vi "AnalyzePulseTrain for PulseGuard.vi"(0 "Waveform In":waveform(dbl)={"t0"=timestamp(3433165898.5470004 s since 1904-01-01), "dt"=1e-05, "Y"=array[4250 elements]}, 5 "Repetitions in the Input Waveform":i32, 7 "Pulse Characteristics":T1={"Pulses per Cycle"=2, "Load Resistance (Ohms)"=750.0, "Krec Value"=2, "Recovery Mode (T=Active)"=TRUE, "Target Stim Currents (Amps)"=[]}) -> (2 "Last Pulse Width":dbl format="%0.2f", 4 "Number of Pulses Found":i32, 8 "Last Pulse Amplitude":dbl format="%0.2f")   [LabVIEW 2010]
uses:
  <vilib>/measure/mamon.llb/Trigger Detection for 1 Channel.vi
  <vilib>/measure/NI_MAPro.lvlib
  <vilib>/Analysis/NI_AALBase.lvlib
panel:
  out "Normalized Waveform":waveform(dbl)(graph)
  # "The input waveform should be a capture of the STIM chip output\n(before the cap) when the output is held at 1/2 HVDD by the\nLoad Resistance.  This ensures that passive recovery and CBC\npulses are captured, because they look like pulses pulled to GND."
  # "The elements in these arrays correspond to the pulses per cycle.\nThey are the averages over all the repetitions in the waveform."
  # "Enter Target Current\nfor each in array below"
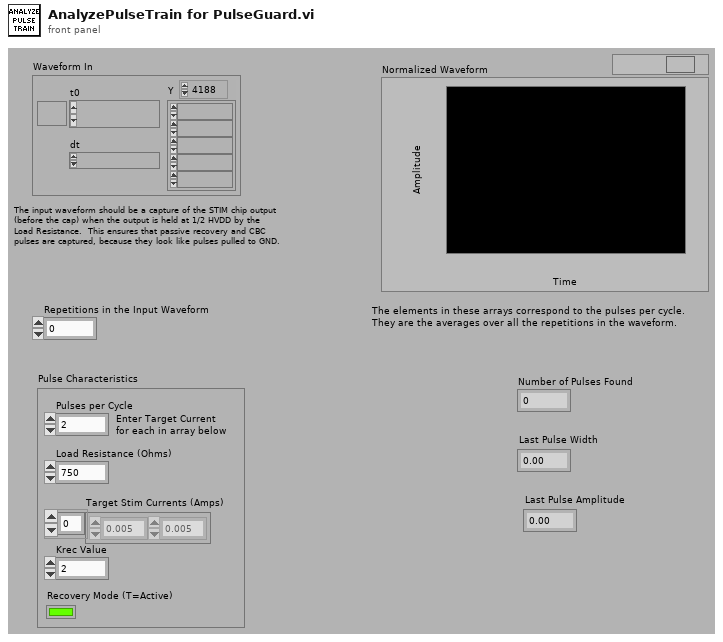
[diagram p1: front panel]
types:
  T1 = cluster{"Pulses per Cycle":i32, "Load Resistance (Ohms)":dbl, "Krec Value":i32, "Recovery Mode (T=Active)":bool, "Target Stim Currents (Amps)":dbl[]}
  T2 = cluster{"trigger slope":u16, "Trigger Level":dbl}[]
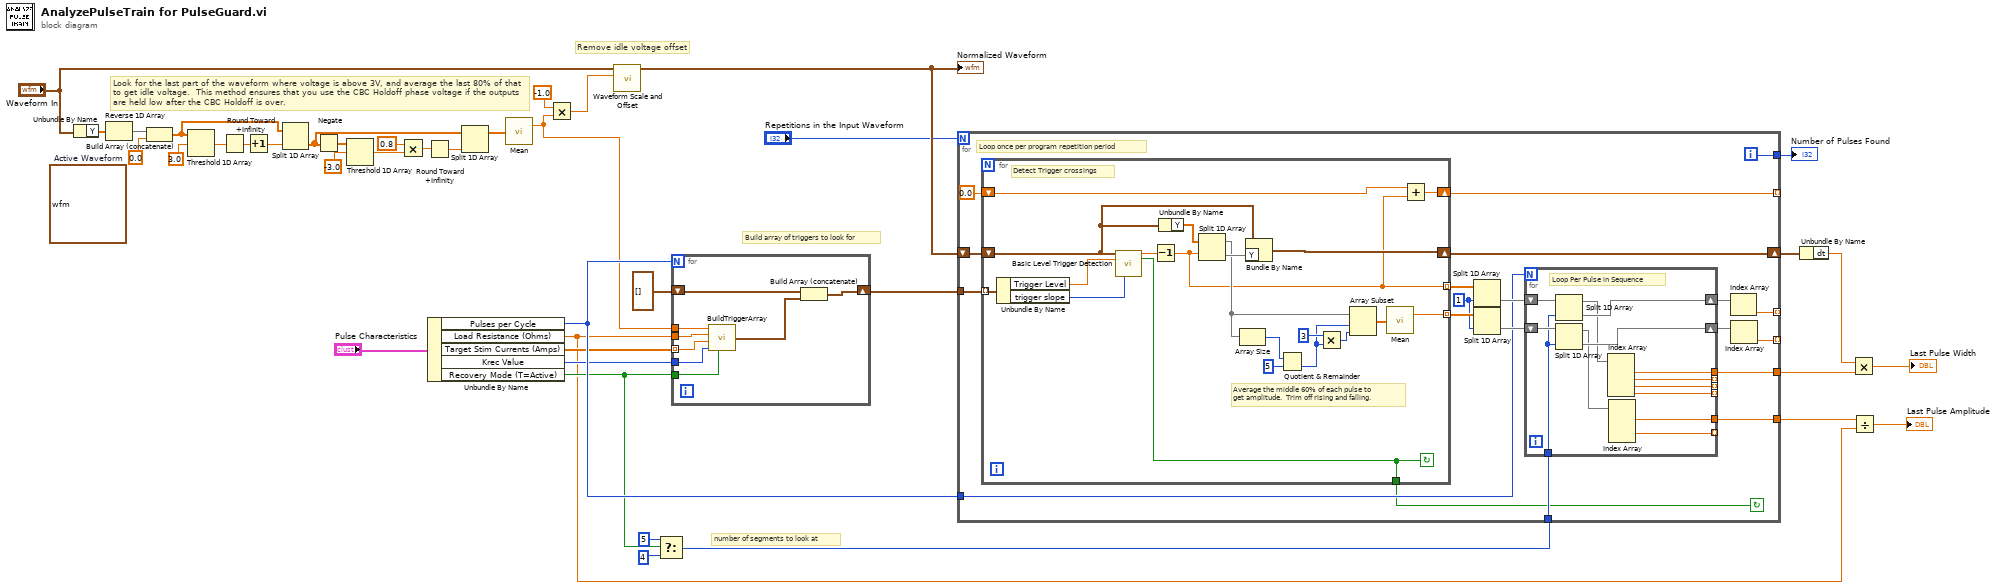
[diagram p0: block diagram]
diagram:
  (unwired) waveform(dbl) {"t0"=timestamp(3418839276.250478 s since 1904-01-01), "dt"=1e-06, "Y"=[5.0, 5.0, 9.0, 9.0, 9.0, 9.0, 9.0, 9.0, 9.0, 9.0, 5.0, 5.0, 5.0, 3.0, 3.0, 3.0, 3.0, 3.0, 3.0, 3.0, 3.0, 3.0, 3.0, 3.0, 3.0, 3.0, 3.0, 3.0, 3.0, 5.0, 5.0, 5.0, 5.0, 8.0, 8.0, 8.0, 8.0, 8.0, 8.0, 8.0, 8.0, 5.0, 5.0, 5.0, 3.0, 3.0, 3.0, 3.0, 3.0, 3.0, 3.0, 3.0, 3.0, 3.0, 3.0, 3.0, 3.0, 3.0, 3.0, 3.0, 5.0, 5.0, 5.0, 5.0, 0.0, 0.0, 0.0, 0.0, 0.0, 5.0, 5.0, 5.0, 5.0, 5.0, 5.0, 5.0, 5.0, 5.0, 5.0, 5.0, 5.0, 5.0, 5.0, 5.0, 5.0, 5.0, 5.0, 5.0, 5.0, 5.0, 5.0, 5.0, 5.0, 5.0, 5.0, 5.0, 5.0, 5.0, 5.0, 5.0, 5.0, 5.0, 9.0, 9.0, 9.0, 9.0, 9.0, 9.0, 9.0, 9.0, 5.0, 5.0, 5.0, 3.0, 3.0, 3.0, 3.0, 3.0, 3.0, 3.0, 3.0, 3.0, 3.0, 3.0, 3.0, 3.0, 3.0, 3.0, 3.0, 5.0, 5.0, 5.0, 5.0, 8.0, 8.0, 8.0, 8.0, 8.0, 8.0, 8.0, 8.0, 5.0, 5.0, 5.0, 3.0, 3.0, 3.0, 3.0, 3.0, 3.0, 3.0, 3.0, 3.0, 3.0, 3.0, 3.0, 3.0, 3.0, 3.0, 3.0, 5.0, 5.0, 5.0, 5.0, 0.0, 0.0, 0.0, 0.0, 0.0, 5.0, 5.0, 5.0, 5.0, 5.0, 5.0, 5.0, 5.0, 5.0, 5.0, 5.0, 5.0, 5.0, 5.0, 5.0, 5.0, 5.0, 5.0, 5.0, 5.0, 5.0, 5.0, 5.0, 5.0, 5.0, 5.0, 5.0, 5.0, 5.0, 5.0, 5.0, 5.0, 5.0, 9.0, 9.0, 9.0, 9.0, 9.0, 9.0, 9.0, 9.0, 5.0, 5.0, 5.0, 3.0, 3.0, 3.0, 3.0, 3.0, 3.0, 3.0, 3.0, 3.0, 3.0, 3.0, 3.0, 3.0, 3.0, 3.0, 3.0, 5.0, 5.0, 5.0, 5.0, 8.0, 8.0, 8.0, 8.0, 8.0, 8.0, 8.0, 8.0, 5.0, 5.0, 5.0, 3.0, 3.0, 3.0, 3.0, 3.0, 3.0, 3.0, 3.0, 3.0, 3.0, 3.0, 3.0, 3.0, 3.0, 3.0, 3.0, 5.0, 5.0, 5.0, 5.0, 0.0, 0.0, 0.0, 0.0, 0.0, 5.0, 5.0, 5.0, 5.0, 5.0, 5.0, 5.0, 5.0, 5.0, 5.0, 5.0, 5.0, 5.0, 5.0, 5.0, 5.0, 5.0, 5.0, 5.0, 5.0, 5.0, 5.0, 5.0, 5.0, 5.0, 5.0, 5.0, 5.0, 5.0, 5.0, 5.0, 5.0, 5.0, 9.0, 9.0, 9.0, 9.0, 9.0, 9.0, 9.0, 9.0, 5.0, 5.0, 5.0, 3.0, 3.0, 3.0, 3.0, 3.0, 3.0, 3.0, 3.0, 3.0, 3.0, 3.0, 3.0, 3.0, 3.0, 3.0, 3.0, 5.0, 5.0, 5.0, 5.0, 8.0, 8.0, 8.0, 8.0, 8.0, 8.0, 8.0, 8.0, 5.0, 5.0, 5.0, 3.0, 3.0, 3.0, 3.0, 3.0, 3.0, 3.0, 3.0, 3.0, 3.0, 3.0, 3.0, 3.0, 3.0, 3.0, 3.0, 5.0, 5.0, 5.0, 5.0, 0.0, 0.0, 0.0, 0.0, 0.0, 5.0, 5.0, 5.0, 5.0, 5.0, 5.0, 5.0, 5.0, 5.0, 5.0, 5.0, 5.0, 5.0, 5.0, 5.0, 5.0, 5.0, 5.0, 5.0, 5.0, 5.0, 5.0, 5.0, 5.0, 5.0, 5.0, 5.0, 5.0, 5.0, 5.0, 5.0, 5.0, 5.0, 9.0, 9.0, 9.0, 9.0, 9.0, 9.0, 9.0, 9.0, 5.0, 5.0, 5.0, 3.0, 3.0, 3.0, 3.0, 3.0, 3.0, 3.0, 3.0, 3.0, 3.0, 3.0, 3.0, 3.0, 3.0, 3.0, 3.0, 5.0, 5.0, 5.0, 5.0, 8.0, 8.0, 8.0, 8.0, 8.0, 8.0, 8.0, 8.0, 5.0, 5.0, 5.0, 3.0, 3.0, 3.0, 3.0, 3.0, 3.0, 3.0, 3.0, 3.0, 3.0, 3.0, 3.0, 3.0, 3.0, 3.0, 3.0, 5.0, 5.0, 5.0, 5.0, 0.0, 0.0, 0.0, 0.0, 0.0, 5.0, 5.0, 5.0, 5.0, 5.0, 5.0, 5.0, 5.0, 5.0, 5.0, 5.0, 5.0, 5.0, 5.0, 5.0, 5.0, 5.0, 5.0, 5.0, 5.0, 5.0, 5.0, 5.0, 5.0, 5.0, 5.0, 5.0, 5.0, 5.0, 5.0, 5.0, 5.0, 5.0, 5.0]}  # Active Waveform
  # "number of segments to look at"
  # "Look for the last part of the waveform where voltage is above 3V, and average the last 80% of that\nto get idle voltage.  This method ensures that you use the CBC Holdoff phase voltage if the outputs\nare held low after the CBC Holdoff is over."
  # "Build array of triggers to look for"
  # "Remove idle voltage offset"
  n1 = Unbundle By Name("Waveform In") -> ("Y"=w29:dbl[])
  n2 = Reverse 1D Array(array=w29) -> (reversed array=w28:dbl[])
  n3 = Build Array (concatenate)(w28, 0.0 ("y")) -> (w23:dbl[])
  n4 = Threshold 1D Array(2:3.0 ("y"), 3:w23) -> (0:w25:dbl)  [unwired: 1 in]
  n5 = Round Toward +Infinity(x=w25) -> (ceil(x): smallest int >= x=w24:dbl)
  n6 = Increment(x=w24) -> (x+1=w14:dbl)
  n7 = Split 1D Array(array=w23, index=w14) -> (second subarray=w16:dbl[])  [unwired: 1 out]
  n8 = Negate(x=w16) -> (-x=w21:dbl[])
  n9 = Threshold 1D Array(2:-3.0 ("y"), 3:w21) -> (0:w20:dbl)  [unwired: 1 in]
  n10 = Multiply(x=0.8, y=w20) -> (x*y=w18:dbl)
  n11 = Round Toward +Infinity(x=w18) -> (ceil(x): smallest int >= x=w17:dbl)
  n12 = Unbundle By Name("Pulse Characteristics") -> ("Pulses per Cycle"=w34:i32, "Load Resistance (Ohms)"=w3:dbl, "Target Stim Currents (Amps)"=w33:dbl[], "Krec Value"=w32:i32, "Recovery Mode (T=Active)"=w11:bool)
  n13 = Split 1D Array(array=w16, index=w17) -> (first subarray=w15:dbl[])  [unwired: 1 out]
  n14 = call <vilib>:"Mean.vi"("X"=w15) -> ("mean"=w12:dbl)  [unwired: 1 out]
  n15 = Multiply(x=-1.0, y=w12) -> (x*y=w36:dbl)
  n16 = call <vilib>:"Waveform Scale and Offset.vi"("offset"=w36, "waveform in"="Waveform In") -> ("waveform out"=w35:waveform(dbl))  [unwired: 8 in, 1 out]
  "Normalized Waveform" <- w35
  n17 = Select(t=5, s=w11, f=4 ("index")) -> (s? t:f=w9:i32)
  n18 = for {
    N: w34 -> [_]
    shift-right: [w48] -> w13
    shift-left: T2 [] -> [w47]
    tunnel: w12 -> [w46]
    tunnel: w11 -> [w45]
    tunnel: w3 -> [w44]
    tunnel: w33 -> [w43] mode=indexing
    tunnel: w32 -> [w42]
    n19 = call "BuildTriggerArray.vi"("CBC Trigger Level"=w46, "Load Resistance (Ohms)"=w44, "Target Stim Current (Amps)"=w43, "Krec Value"=w42, "Recovery Mode (T=Active)"=w45) -> ("Pulse Triggers"=w41:T2)
    n20 = Build Array (concatenate)(w47, w41) -> (w48:T2)
  }
  n21 = for {
    N: "Repetitions in the Input Waveform" -> [_]
    tunnel: w13 -> [w68]
    shift-right: [w64] -> w30
    shift-left: w35 -> [w67]
    tunnel: w34 -> [w61]
    tunnel: [w58] -> _ mode=indexing
    tunnel: [w57] -> _ mode=indexing
    tunnel: [w54] -> _ mode=indexing
    tunnel: w9 -> [w53]
    tunnel: [w52] -> w7
    tunnel: [w50] -> w6
    tunnel: [w49] -> w4
    i -> [w52]
    stop <- w51 continue-if-true
    w65 = 1 ("index")
    # "Loop once per program repetition period"
    n22 = for {
      tunnel: w68 -> [w101] mode=indexing
      shift-right: [w87] -> w64
      shift-left: w67 -> [w96]
      tunnel: [w88] -> w66 mode=indexing
      tunnel: [w83] -> w55 mode=indexing
      shift-right: [w86] -> w54
      shift-left: 0.0 -> [w85]
      tunnel: [w82] -> w51
      stop <- w82 continue-if-true
      # "Detect Trigger crossings"
      # "Average the middle 60% of each pulse to\nget amplitude.  Trim off rising and falling."
      n23 = Unbundle By Name(w101) -> ("Trigger Level"=w100:dbl, "trigger slope"=w99:u16)
      n24 = call-poly <vilib>:"Basic Level Trigger Detection.vi"("signal in"=w96, "level"=w100, "trigger slope"=w99) -> ("trigger location"=w84:dbl, "trigger detected?"=w82:bool)  [unwired: 10 in, 1 out]
      n25 = Decrement(x=w84) -> (x-1=w83:dbl)
      n26 = Unbundle By Name(w96) -> ("Y"=w98:dbl[])
      n27 = Split 1D Array(array=w98, index=w83) -> (first subarray=w90:dbl[], second subarray=w97:dbl[])
      n28 = Array Size(array=w90) -> (size(s)=w95:i32)
      n29 = Bundle By Name(cluster=w96, "Y"=w97) -> (w87:waveform(dbl))
      n30 = Quotient & Remainder(x=w95, y=5) -> (floor(x/y)=w92:i32)  [unwired: 1 out]
      n31 = Multiply(x=3, y=w92) -> (x*y=w91:i32)
      n32 = Array Subset(array=w90, index=w92, length=w91) -> (w89:dbl[])
      n33 = call <vilib>:"Mean.vi"("X"=w89) -> ("mean"=w88:dbl)  [unwired: 1 out]
      n34 = Add(x=w85, y=w83) -> (x+y=w86:dbl)
    }
    n35 = Split 1D Array(array=w55, index=w65) -> (second subarray=w63:dbl[])  [unwired: 1 out]
    n36 = Split 1D Array(array=w66, index=w65) -> (second subarray=w62:dbl[])  [unwired: 1 out]
    n37 = for {
      N: w61 -> [_]
      shift-right: [w79] -> w60
      shift-left: w63 -> [w81]
      shift-right: [w78] -> w59
      shift-left: w62 -> [w80]
      tunnel: [w75] -> w50
      tunnel: [w74] -> _ mode=indexing
      tunnel: [w73] -> _ mode=indexing
      tunnel: [w72] -> _ mode=indexing
      tunnel: [w71] -> w49
      tunnel: [w70] -> _ mode=indexing
      tunnel: w53 -> [w69]
      # "Loop Per Pulse in Sequence"
      n38 = Split 1D Array(array=w81, index=w69) -> (first subarray=w77:dbl[], second subarray=w79:dbl[])
      n39 = Split 1D Array(array=w80, index=w69) -> (first subarray=w76:dbl[], second subarray=w78:dbl[])
      n40 = Index Array(array=w77) -> (element #1=w75:dbl, element #2=w74:dbl, element #3=w73:dbl, element #4=w72:dbl)  [unwired: 4 in]
      n41 = Index Array(array=w76) -> (element #1=w71:dbl, element #3=w70:dbl)  [unwired: 4 in, 2 out]
    }
    n42 = Index Array(array=w60) -> (element=w58:dbl)  [unwired: 1 in]
    n43 = Index Array(array=w59) -> (element=w57:dbl)  [unwired: 1 in]
  }
  "Number of Pulses Found" <- w7
  n44 = Unbundle By Name(w30) -> ("dt"=w5:dbl)
  n45 = Multiply(x=w5, y=w6) -> (x*y=→"Last Pulse Width":dbl)
  n46 = Divide(x=w4, y=w3) -> (x/y=→"Last Pulse Amplitude":dbl)
